vi "C Series Module Information (Scan Interface).vi"(8 "error in":errorcluster, 10 "Number of Slots":i32, 11 "Address (localhost)":string) -> (0 "error out":errorcluster, 2 "Module information":T1[](array[typedef]) {"Module Code" format="%.0x"})   [LabVIEW 2015, in "SMI.lvlib" / "C Series Module.lvclass"]
uses:
  C Series Module.lvclass
  Module/Controls/ModuleInformation.ctl
  <vilib>/regexp/Match Regular Expression.xnode
  <resource>/objmgr/ni.var.rc
  Module/Module.lvclass
  <resource>/objmgr/cRIO.rc
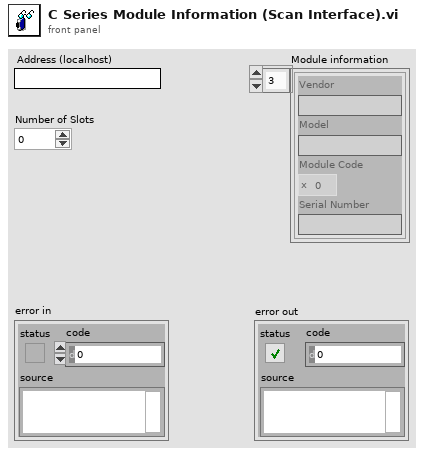
[diagram p1: front panel]
types:
  T1 = typedef "SMI.lvlib/Module.lvclass/ModuleInformation.ctl" = cluster{"Vendor":string, "Model":string, "Module Code":u16, "Serial Number":string}
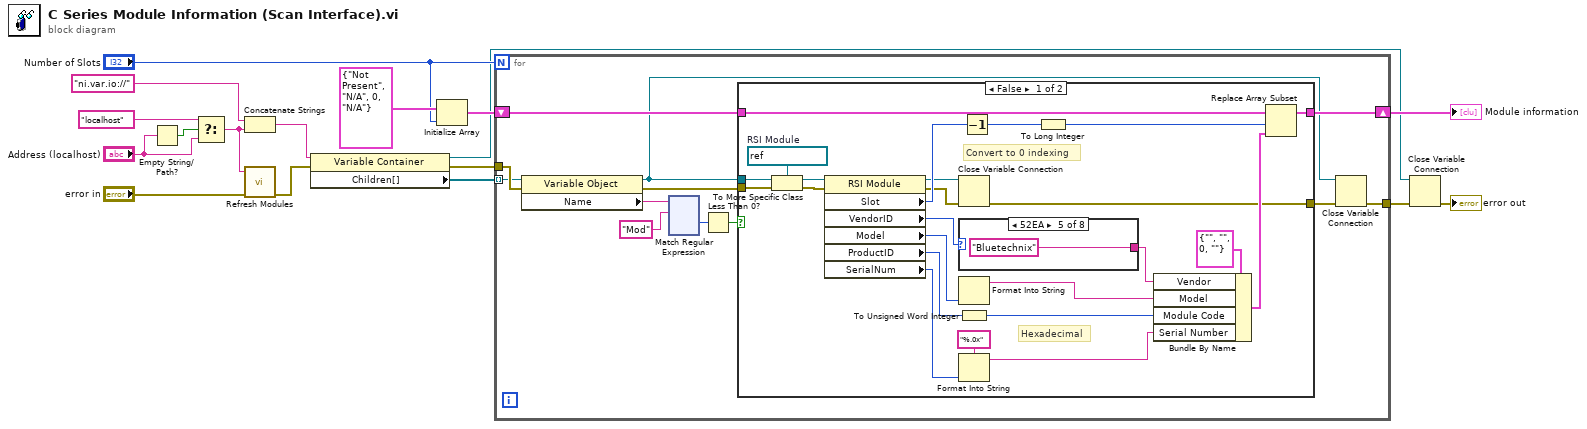
[diagram p0: block diagram]
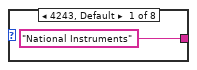
[diagram p2: hidden frame]
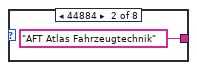
[diagram p3: hidden frame]
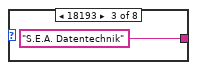
[diagram p4: hidden frame]
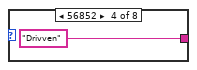
[diagram p5: hidden frame]
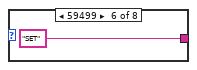
[diagram p6: hidden frame]
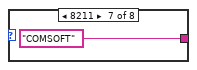
[diagram p7: hidden frame]
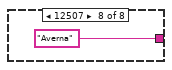
[diagram p8: hidden frame]
diagram:
  n1 = Empty String/Path?(string/path="Address (localhost)") -> (empty?=w13:bool)
  n2 = Select(t="localhost" ("Resource 2"), s=w13, f="Address (localhost)") -> (s? t:f=w9:string)
  n3 = Concatenate Strings("ni.var.io://" ("Resource 2"), w9) -> (w8:string)
  n4 = call <vilib>:"Refresh Modules.vi"("error in (no error)"="error in", "target address (localhost)"=w9) -> ("error out"=w14:errorcluster)  [unwired: 9 in]
  n5 = property class="Variable Container"(reference=w8, error in=w14) -> (reference out=w4:refnum<k21>, error out=w15:errorcluster, "Children[]"=w3:refnum<k21>[])
  n6 = Initialize Array(T1 {"Vendor"="Not Present", "Model"="N/A", "Module Code"=0, "Serial Number"="N/A"} ("cRIO Module Information"), "Number of Slots") -> (w5:T1[])
  n7 = for {
    N: "Number of Slots" -> [_]
    tunnel: w3 -> [w21] mode=indexing
    tunnel: w15 -> [w23]
    tunnel: [w19] -> w1
    shift-right: [w26] -> w17
    shift-left: w5 -> [w25]
    n8 = property class="Variable Object"(reference=w21, error in=w23) -> (reference out=w20:refnum<k21>, error out=w22:errorcluster, "Name"=w27:string)
    n9 = xnode "Match Regular Expression"("input string"=w27, "regular expression"="Mod") -> ("offset past match"=w29:i32)  [unwired: 4 in, 4 out]
    n10 = Less Than 0?(x=w29) -> (x < 0?=w24:bool)
    n11 = case shown="False" w24 {
      tunnel: w22 -> [w52 w62]
      tunnel: w20 -> [w51 _]
      tunnel: [w40 w62] -> w18
      tunnel: [w50 w63] -> w26
      tunnel: w25 -> [w49 w63]
      frame False {
        w53 = refnum<k21> refnum  # RSI Module
        # "Hexadecimal"
        # "Convert to 0 indexing"
        n12 = To More Specific Class(target class=w53, reference=w51, error in=w52) -> (specific class reference=w48:refnum<k21>, error out=w47:errorcluster)
        n13 = property class="RSI Module"(reference=w48, error in=w47) -> (reference out=w42:refnum<k21>, error out=w41:errorcluster, "Slot"=w45:u32, "VendorID"=w38:u32, "Model"=w36:u32, "ProductID"=w34:u32, "SerialNum"=w32:u32)
        n14 = Close Variable Connection(8:w41, 11:w42) -> (0:w40:errorcluster)
        n15 = case shown="52EA" w38 {
          tunnel: ["National Instruments" "AFT Atlas Fahrzeugtechnik" "S.E.A. Datentechnik" "Drivven" "Bluetechnix" "SET" "COMSOFT" "Averna"] -> w37
          frame 4243, Default {
          }
          frame 44884 {
          }
          frame 18193 {
          }
          frame 56852 {
          }
          frame 21226 {
          }
          frame 59499 {
          }
          frame 8211 {
          }
          frame 12507 {
          }
        }
        n16 = Format Into String(w36) -> (resulting string=w35:string)  [unwired: 3 in, 1 out]
        n17 = To Unsigned Word Integer(number=w34) -> (unsigned 16bit integer=w33:u16)
        n18 = Format Into String(format string="%.0x", w32) -> (resulting string=w31:string)  [unwired: 2 in, 1 out]
        n19 = Decrement(x=w45) -> (x-1=w39:u32)
        n20 = To Long Integer(number=w39) -> (32bit integer=w44:i32)
        n21 = Bundle By Name(cluster=T1 {"Vendor"="", "Model"="", "Module Code"=0, "Serial Number"=""} ("cRIO Module Information"), "Vendor"=w37, "Model"=w35, "Module Code"=w33, "Serial Number"=w31) -> (w43:T1)
        n22 = Replace Array Subset(array=w49, new element=w43, index=w44) -> (w50:T1[])
      }
      frame True {
        # "The Variable Object is not a module"
      }
    }
    n23 = Close Variable Connection(8:w18, 11:w20) -> (0:w19:errorcluster)
  }
  "Module information" <- w17
  n24 = Close Variable Connection(8:w1, 11:w4) -> (0:→"error out":errorcluster)
